vi "LoopThroughControls.vi"() -> ()   [LabVIEW 2019]
panel:
  in  "Numeric 5":dbl
  in  "Numeric 4":dbl
  out "Control Array":string[](array[string])
  in  "Numeric 3":dbl
  in  "Numeric 2":dbl
  in  "Numeric":dbl
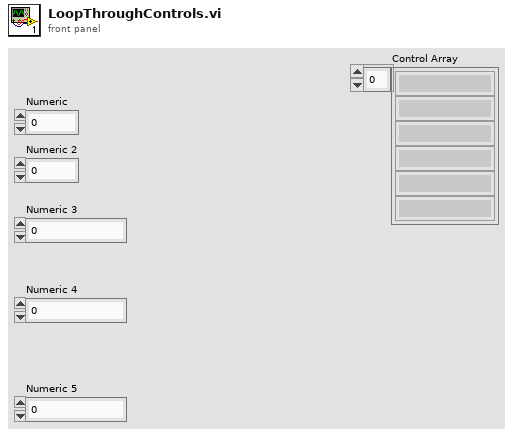
[diagram p1: front panel]
types:
  T1 = enum16{"open", "replace", "create", "open or create", "replace or create", "replace or create with confirmation"}
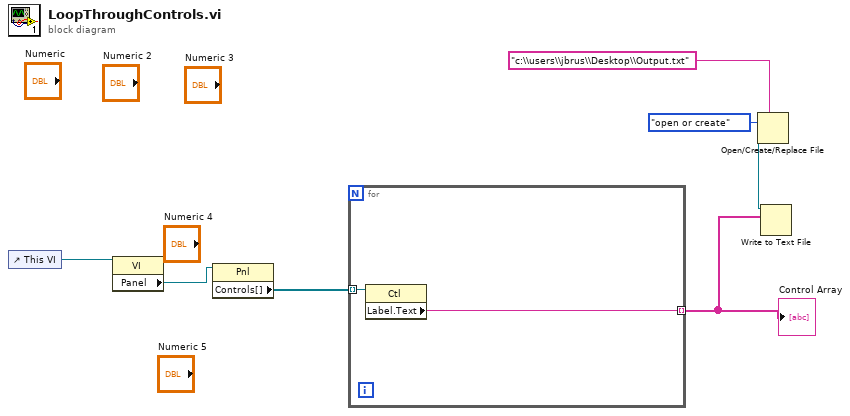
[diagram p0: block diagram]
diagram:
  n1 = control-ref of="This VI"() -> (w7:refnum<vi>)
  n2 = property class="VI"(reference=w7) -> ("Panel"=w6:refnum<vi>)  [unwired: 1 in, 2 out]
  n3 = property class="Pnl"(reference=w6) -> ("Controls[]"=w5:refnum<vi>[])  [unwired: 1 in, 2 out]
  n4 = for {
    tunnel: w5 -> [w9] mode=indexing
    tunnel: [w8] -> w4 mode=indexing
    n5 = property class="Ctl"(reference=w9) -> ("Label.Text"=w8:string)  [unwired: 1 in, 2 out]
  }
  "Control Array" <- w4
  n6 = Open/Create/Replace File(prompt="c:\\users\\jbrus\\Desktop\\Output.txt" ("prompt (Choose or enter file path)"), operation (0:open)=T1."open or create") -> (refnum out=w1:refnum<file>)  [unwired: 4 in, 2 out]
  n7 = Write to Text File(file (use dialog)=w1, text=w4) -> ()  [unwired: 2 in, 3 out]
